vi "Comparison By Given Name.vi"(10 "Person B":T1={"ID"=0, "Family Name"="Doe", "Given Name"="John", "Birth Date"=timestamp(3533142714.9178333 s since 1904-01-01)} {"Birth Date" format="%<%Y/%b/%d>T"}, 11 "Person A":T1={"ID"=0, "Family Name"="Smith", "Given Name"="John", "Birth Date"=timestamp(3533056306.0488334 s since 1904-01-01)} {"Birth Date" format="%<%Y/%b/%d>T"}) -> (3 "Swap?":bool)   [LabVIEW 2023]
doc: "This VI says that the two values should swap if Person A has a later birthday. If they have the same birthday, then they should swap if Person A has an alphabetically later name than Person B, checking last name first and then first name."
uses:
  Person Information.ctl
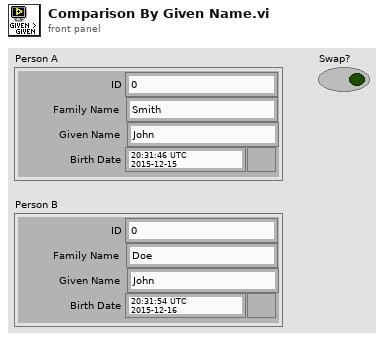
[diagram p1: front panel]
types:
  T1 = typedef "Person Information.ctl" = cluster{"ID":u32, "Family Name":string, "Given Name":string, "Birth Date":timestamp}
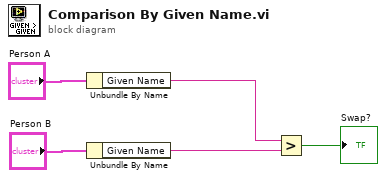
[diagram p0: block diagram]
diagram:
  n1 = Unbundle By Name("Person A") -> ("Given Name"=w3:string)
  n2 = Unbundle By Name("Person B") -> ("Given Name"=w2:string)
  n3 = Greater?(x=w3, y=w2) -> (0:→"Swap?":bool)
